vi "Predator.vi"   [LabVIEW 2017]
panel:
  # "VER1"
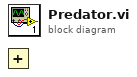
[diagram p0: block diagram]
diagram:
  n1 = Add() -> ()  [unwired: 2 in, 1 out]
